vi "test.vi"() -> (0 "error out":errorcluster)   [LabVIEW 2010, in "Notebook.lvclass"]
uses:
  Notebook.lvclass
panel:
  in  "notebook folder path path":path
  in  "clear":bool
  in  "stop":bool
  in  "insert":bool
  in  "Insert string":string
  in  "notebook":string
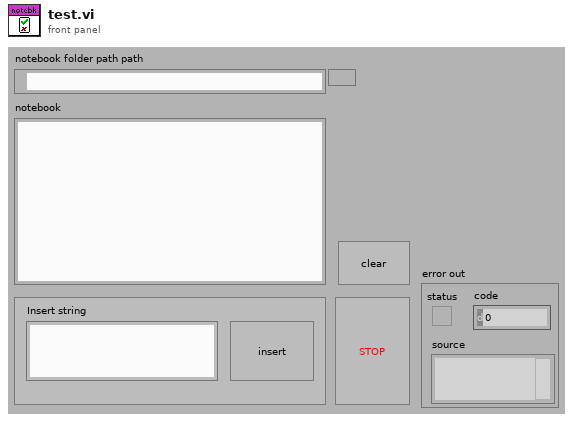
[diagram p1: front panel]
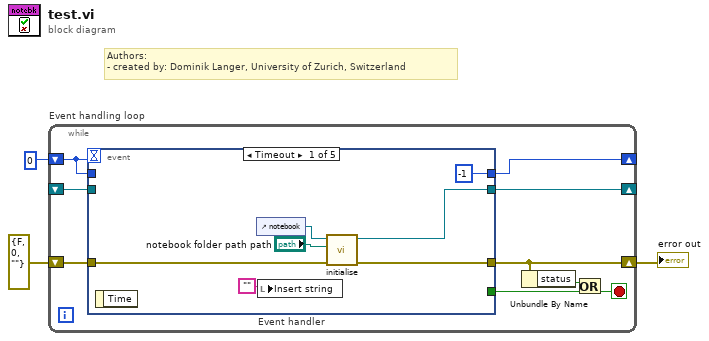
[diagram p0: block diagram]
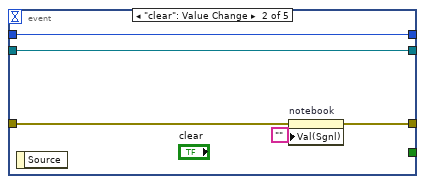
[diagram p2: hidden frame]
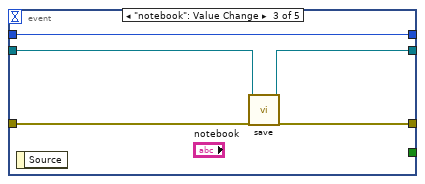
[diagram p3: hidden frame]
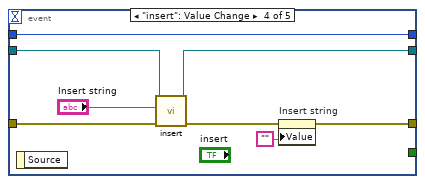
[diagram p4: hidden frame]
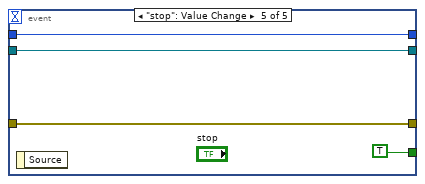
[diagram p5: hidden frame]
diagram:
  # "Authors: \n- created by: Dominik Langer, University of Zurich, Switzerland"
  n1 = while "Event handling loop" {
    shift-right: [w11] -> _
    shift-left: 0 -> [w12]
    shift-right: [w7] -> w2
    shift-left: errorcluster {"status"=FALSE, "code"=0, "source"=""} ("error out") -> [w10]
    shift-right: [w9] -> _
    shift-left: _ -> [w8]
    stop <- w4 stop-if-true
    n2 = event "Event handler" shown="[0] Timeout" {
      selector: _ -> [_ _ _ _ _]
      dyn-events: _ -> [_ _ _ _ _]
      timeout: w12 -> [_ _ _ _ _]
      tunnel: w12 -> [_ w24 w29 w37 w41]
      tunnel: [-1 w24 w29 w37 w41] -> w11
      tunnel: [w13 w22 w27 w31 w40] -> w7
      tunnel: w10 -> [w17 w20 w28 w35 w40]
      tunnel: [w14 w21 w25 w33 w39] -> w9
      tunnel: w8 -> [_ w21 w26 w34 w39]
      tunnel: [_ _ _ _ TRUE] -> w6
      event Timeout {
        n3 = event-data() -> ()  [unwired: 2 out]
        n4 = control-ref of="notebook"() -> (w16:refnum<vi>)
        n5 = local write "Insert string"("") -> ()
        n6 = call "initialise.vi"("error in (no error)"=w17, "folder path"="notebook folder path path", "notebook control ref"=w16) -> ("error out"=w13:errorcluster, "Notebook out"=w14:refnum<class "Notebook.lvclass">)  [unwired: 7 out]
      }
      event "clear": Value Change {
        n7 = event-data() -> ()  [unwired: 2 out]
        n8 = property on="notebook" class="Str"(error in=w20, "Val(Sgnl)"="") -> (error out=w22:errorcluster)  [unwired: 1 in, 1 out]
      }
      event "notebook": Value Change {
        n9 = event-data() -> ()  [unwired: 2 out]
        n10 = call "save.vi"("error in (no error)"=w28, "Notebook in"=w26) -> ("error out"=w27:errorcluster, "Notebook out"=w25:refnum<class "Notebook.lvclass">)  [unwired: 8 out]
      }
      event "insert": Value Change {
        n11 = event-data() -> ()  [unwired: 2 out]
        n12 = call "insert.vi"("error in (no error)"=w35, "string"="Insert string", "Notebook in"=w34) -> ("error out"=w32:errorcluster, "Notebook out"=w33:refnum<class "Notebook.lvclass">)  [unwired: 2 in, 5 out]
        n13 = property on="Insert string" class="Str"(error in=w32, "Value"="") -> (error out=w31:errorcluster)  [unwired: 1 in, 1 out]
      }
      event "stop": Value Change {
        n14 = event-data() -> ()  [unwired: 2 out]
      }
    }
    n15 = Unbundle By Name(w7) -> ("status"=w5:bool)
    n16 = Or(x=w5, y=w6) -> (x .or. y?=w4:bool)
  }
  "error out" <- w2
